vi "Management Object Value to Array of Strings.vi"(3 ".NET Refnum in":refnum<k24>, 4 "error in":errorcluster) -> (0 ".NET Array Ref":refnum<k24>, 1 "error out":errorcluster, 5 "Spreadsheet string":string, 6 "Strings[]":string[](array[string]))   [LabVIEW 2016]
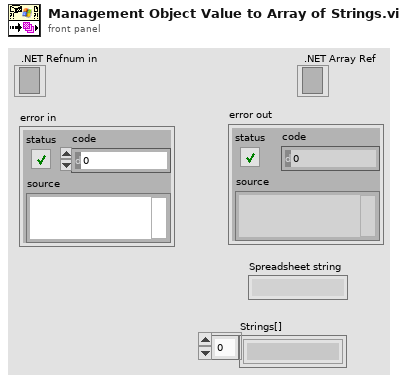
[diagram p1: front panel]
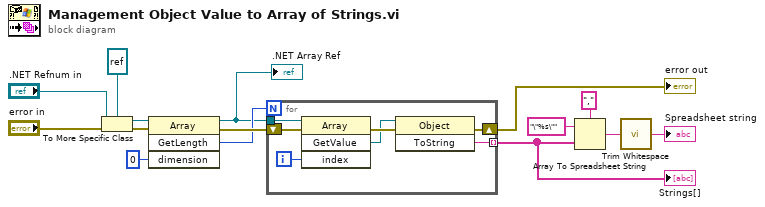
[diagram p0: block diagram]
diagram:
  n1 = To More Specific Class(target class=refnum<k24> refnum ("reference"), reference=".NET Refnum in", error in="error in") -> (specific class reference=w7:refnum<k24>, error out=w10:errorcluster)
  n2 = invoke class="Array" method="GetLength"(reference=w7, error in=w10, "dimension"=0) -> (reference out=w3:refnum<k24>, error out=w11:errorcluster, "GetLength"=w9:i32)  [unwired: 1 in, 1 out]
  ".NET Array Ref" <- w3
  n3 = for {
    N: w9 -> [_]
    tunnel: w3 -> [w20]
    tunnel: [w17] -> w2 mode=indexing
    shift-right: [w16] -> w1
    shift-left: w11 -> [w19]
    i -> [w18]
    n4 = invoke class="Array" method="GetValue"(reference=w20, error in=w19, "index"=w18) -> (error out=w22:errorcluster, "GetValue"=w21:refnum<k24>)  [unwired: 1 in, 2 out]
    n5 = invoke class="Object" method="ToString"(reference=w21, error in=w22) -> (error out=w16:errorcluster, "ToString"=w17:string)  [unwired: 1 in, 1 out]
  }
  "error out" <- w1
  "Strings[]" <- w2
  n6 = Array To Spreadsheet String(delimiter (Tab)=",", array=w2, 3:"\"%s\"" ("format string")) -> (spreadsheet string=w14:string)
  n7 = call <vilib>:"Trim Whitespace.vi"("string"=w14) -> ("trimmed string"=→"Spreadsheet string":string)  [unwired: 1 in]
